vi "dfd_Halfband Filter Design Positive Equiripple TF Modify.vi"(8 "error in (no error)":errorcluster, 10 "actual ripples":dbl[](array[numeric]), 11 "h in":dbl[](array[numeric])) -> (0 "error out":errorcluster, 2 "order out":i32, 3 "h out":dbl[](array[numeric]))   [LabVIEW 2017, in "NI_DigFilter_Process.lvlib"]
uses:
  <vilib>/addons/Digital Filter Design/NI_DigFilter_Process.lvlib
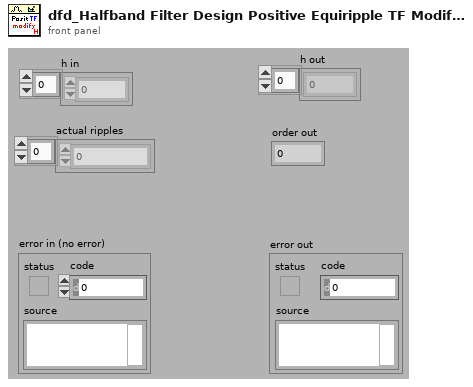
[diagram p1: front panel]
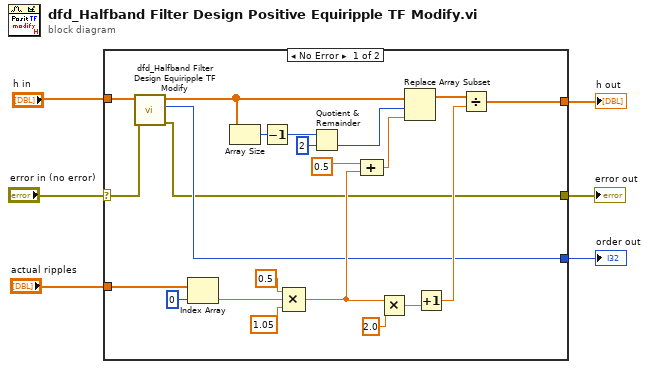
[diagram p0: block diagram]
diagram:
  n1 = case shown="No Error" "error in (no error)" {
    selector: "error in (no error)" -> [w8 w29]
    tunnel: "actual ripples" -> [w24 _]
    tunnel: "h in" -> [w17 _]
    tunnel: [w9 _] -> w2
    tunnel: [w7 w29] -> w3
    tunnel: [w11 _] -> w1
    frame No Error {
      n2 = call <vilib>:"dfd_Halfband Filter Design Equiripple TF Modify.vi"("error in (no error)"=w8, "h in"=w17) -> ("error out"=w7:errorcluster, "order out"=w11:i32, "h out"=w10:dbl[])  [unwired: 1 in, 6 out]
      n3 = Index Array(array=w24, index=0) -> (element=w21:dbl)
      n4 = Array Size(array=w10) -> (size(s)=w26:i32)
      n5 = Decrement(x=w26) -> (x-1=w25:i32)
      n6 = Compound Arithmetic op=MULTIPLY(0.5 ("value"), w21, 1.05 ("y")) -> (w19:dbl)
      n7 = Quotient & Remainder(x=w25, y=2) -> (floor(x/y)=w23:i32)  [unwired: 1 out]
      n8 = Compound Arithmetic op=ADD(0.5 ("value"), w19) -> (w28:dbl)
      n9 = Multiply(x=w19, y=2.0) -> (x*y=w14:dbl)
      n10 = Replace Array Subset(array=w10, new element=w28, index=w23) -> (w16:dbl[])
      n11 = Increment(x=w14) -> (x+1=w18:dbl)
      n12 = Divide(x=w16, y=w18) -> (x/y=w9:dbl[])
    }
    frame Error {
    }
  }
  "error out" <- w3
  "h out" <- w2
  "order out" <- w1
